vi "OP500Z8_PV generator OP100ZENPlus.vi"(6 "3P4S?":bool, 8 "errin":errorcluster, 10 "network":path, 11 "path in":path) -> (0 "sortie d'erreur":errorcluster caption="errout", 2 "network out":path, 3 "tout bon":bool)   [LabVIEW 2020]
uses:
  <vilib>/regexp/Match Regular Expression.xnode
panel:
  out "nombre de remplacements":i32
  out "Chaîne":string
  out "tableau":string[][](array[string])
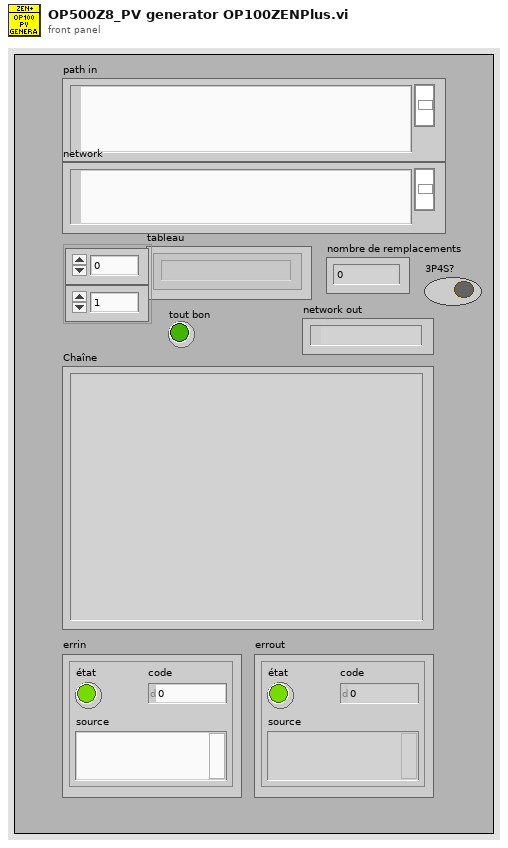
[diagram p1: front panel]
types:
  T1 = enum16{"open", "replace", "create", "open or create", "replace or create", "replace or create with confirmation"}
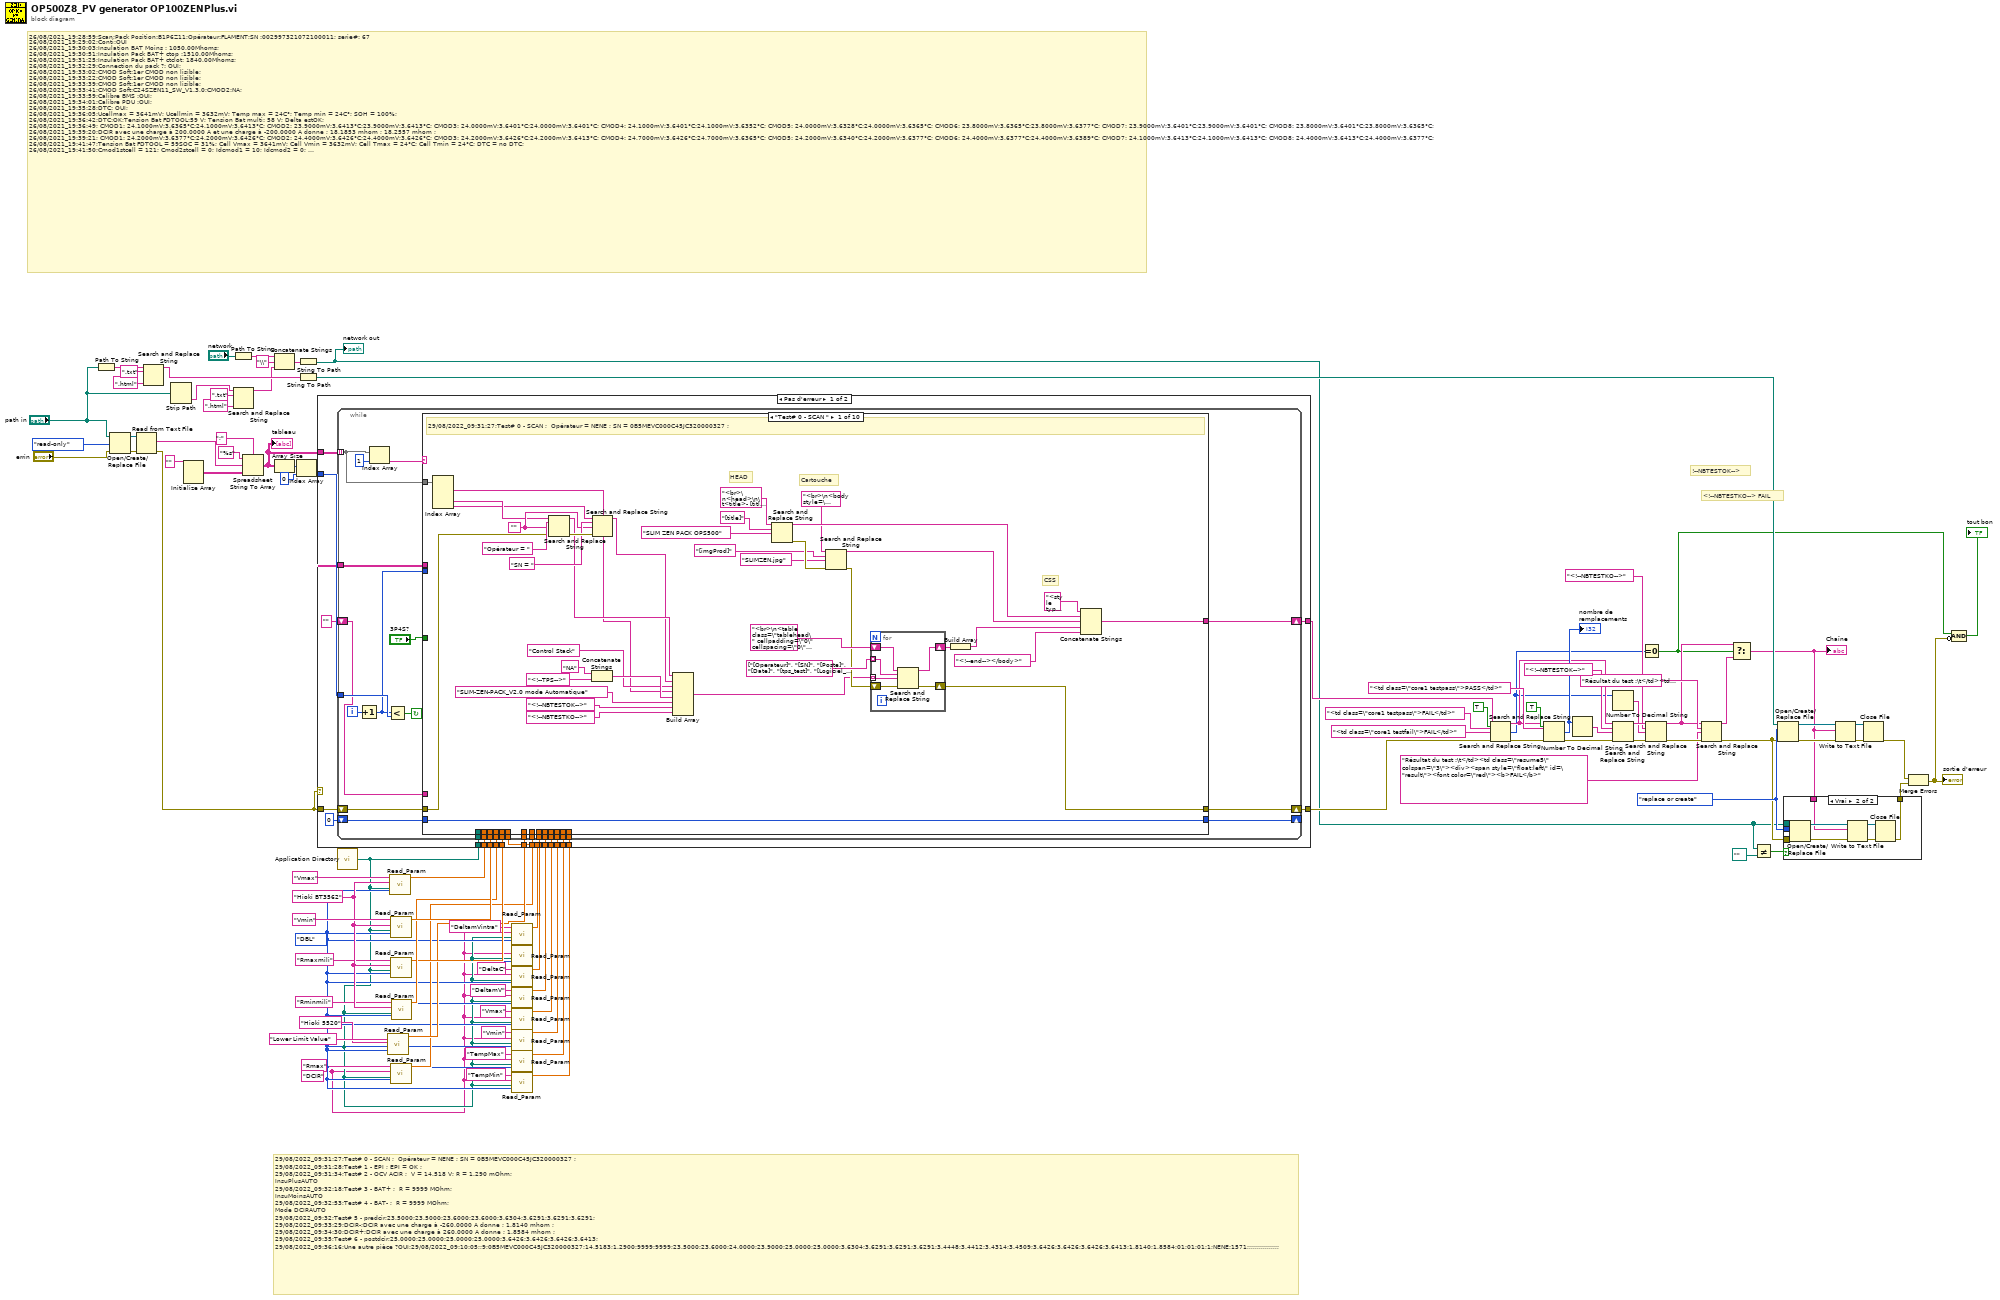
[diagram p0: block diagram]
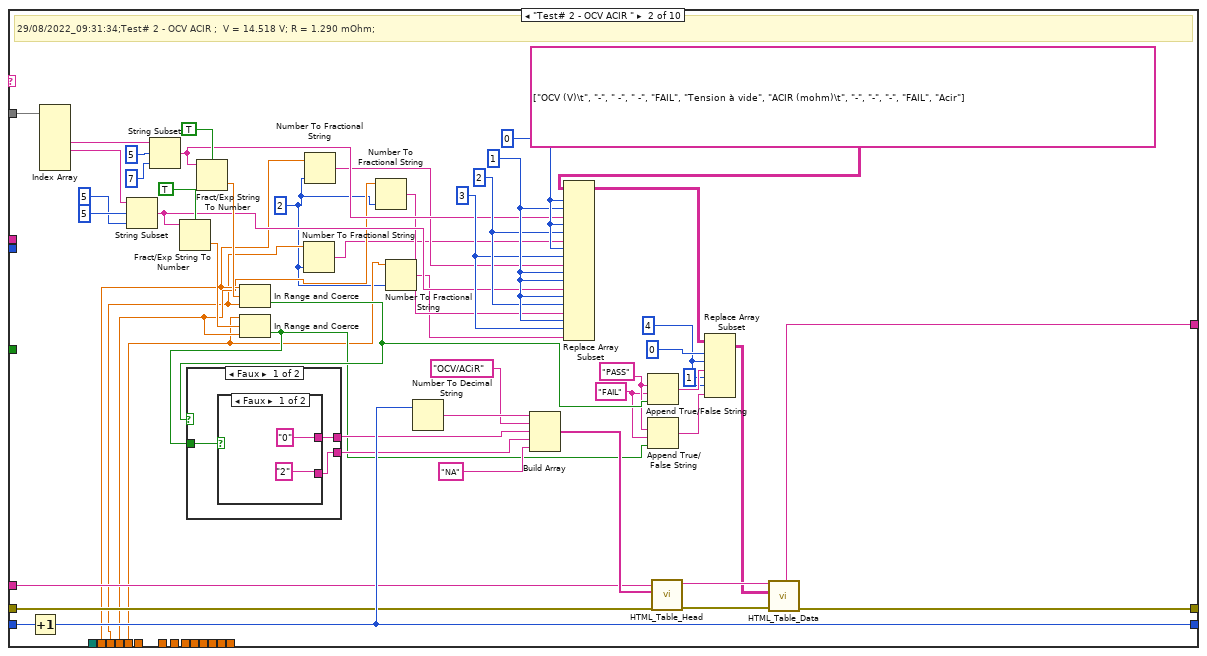
[diagram p2: hidden frame]
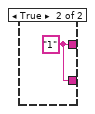
[diagram p3: hidden frame]
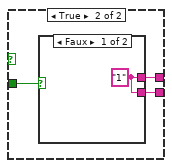
[diagram p4: hidden frame]
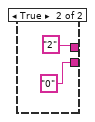
[diagram p5: hidden frame]
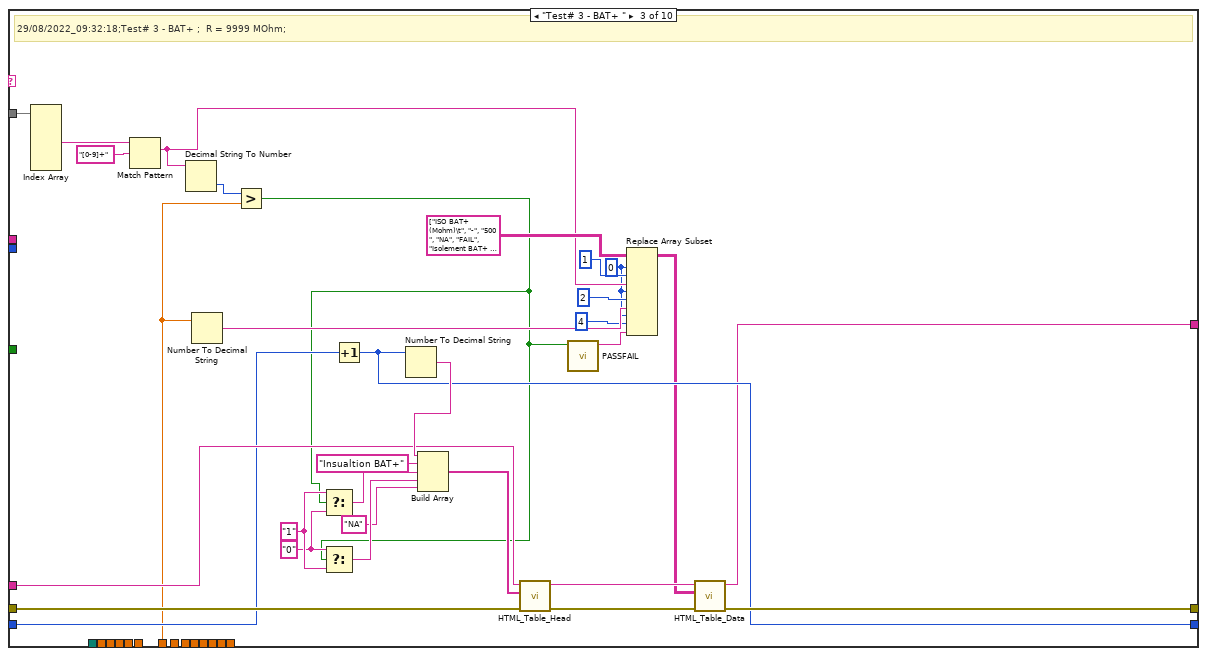
[diagram p6: hidden frame]
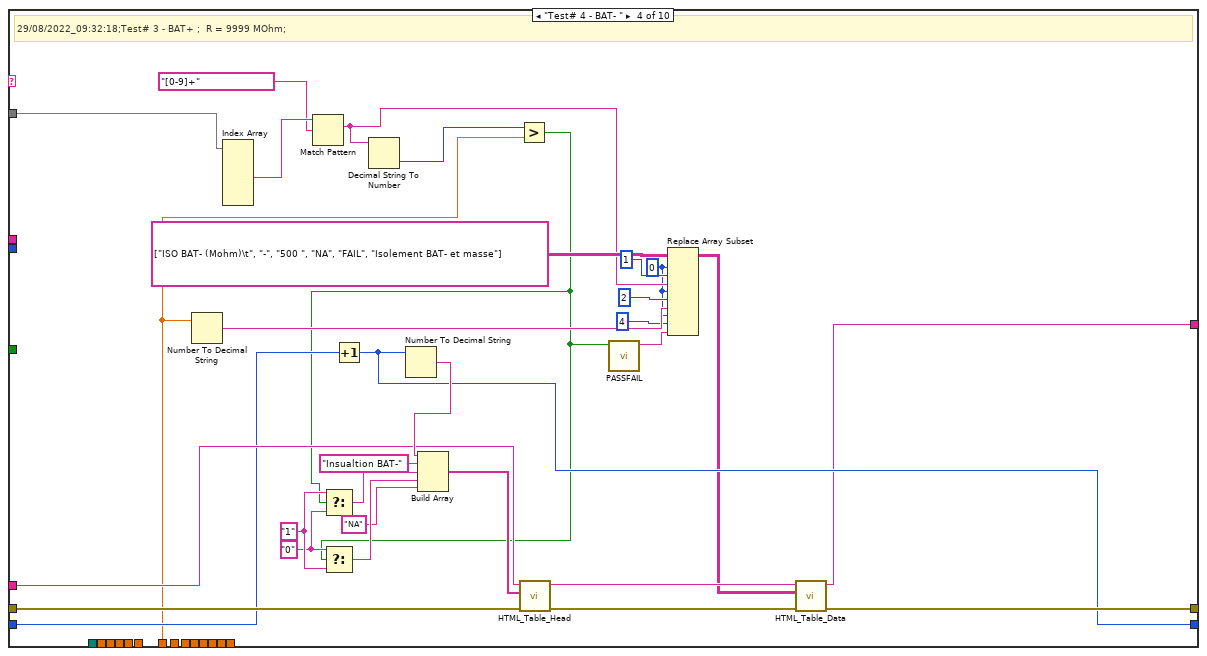
[diagram p7: hidden frame]
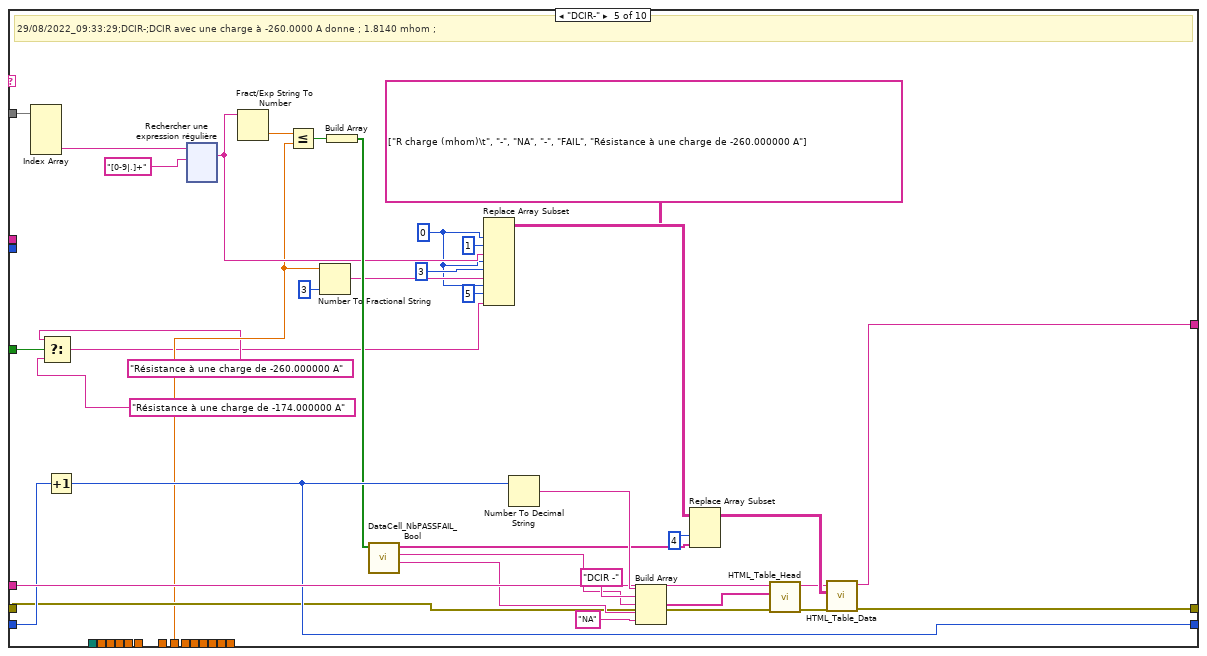
[diagram p8: hidden frame]
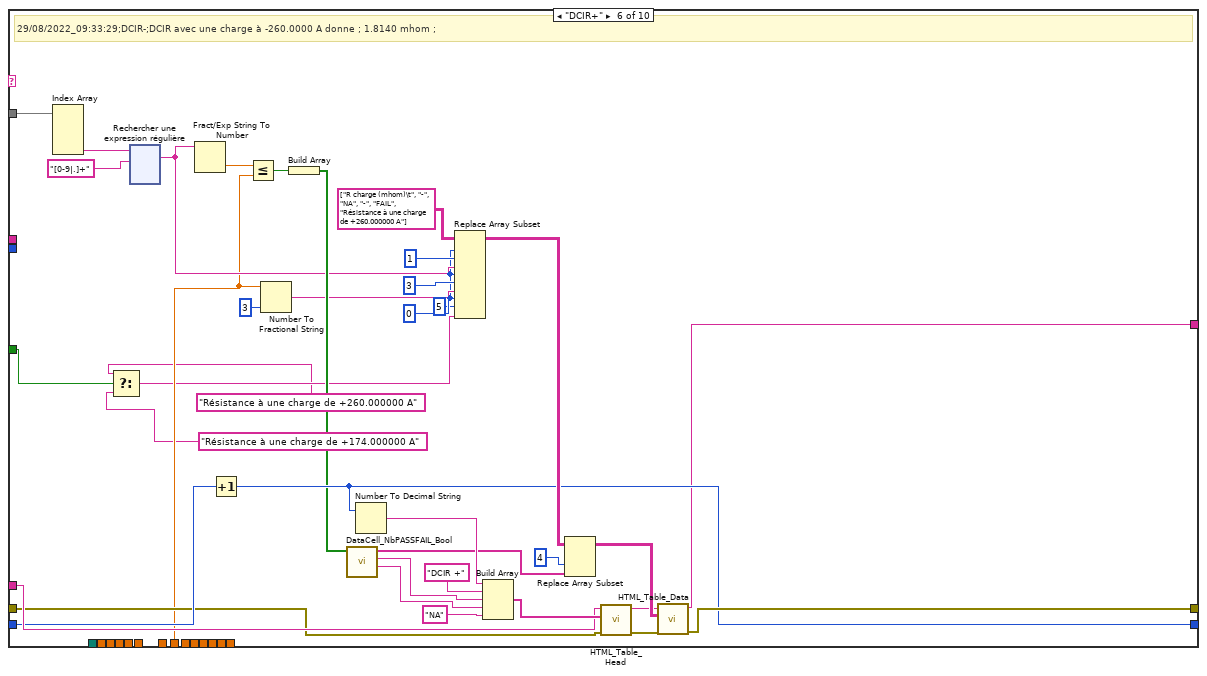
[diagram p9: hidden frame]
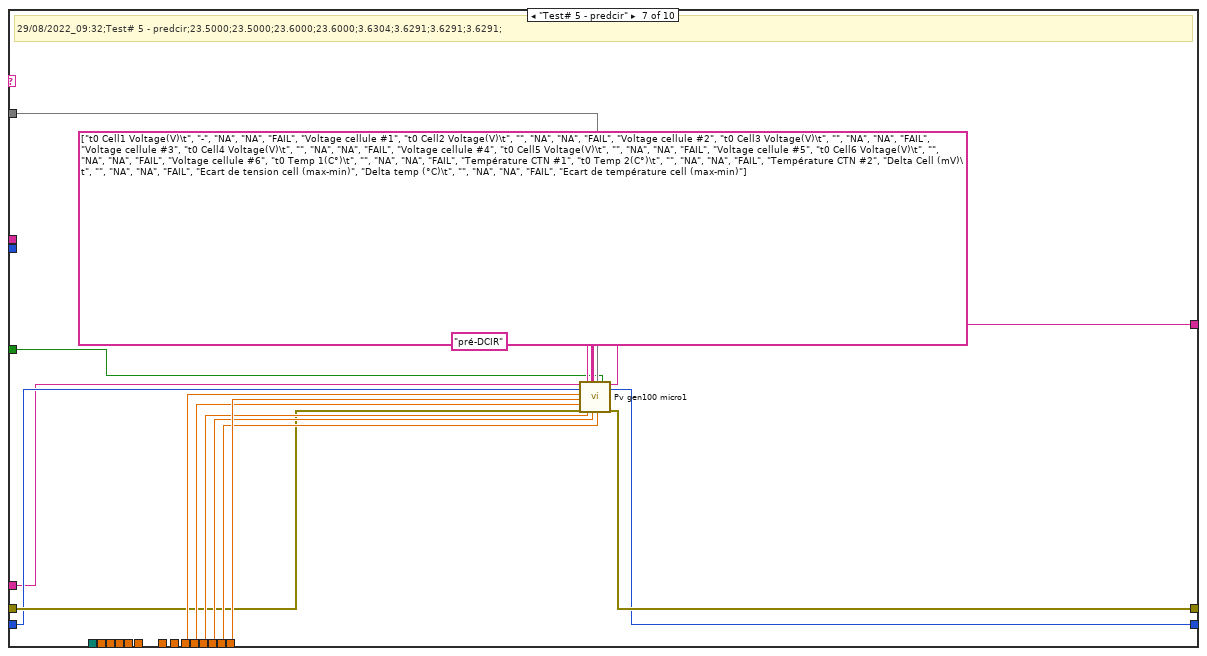
[diagram p10: hidden frame]
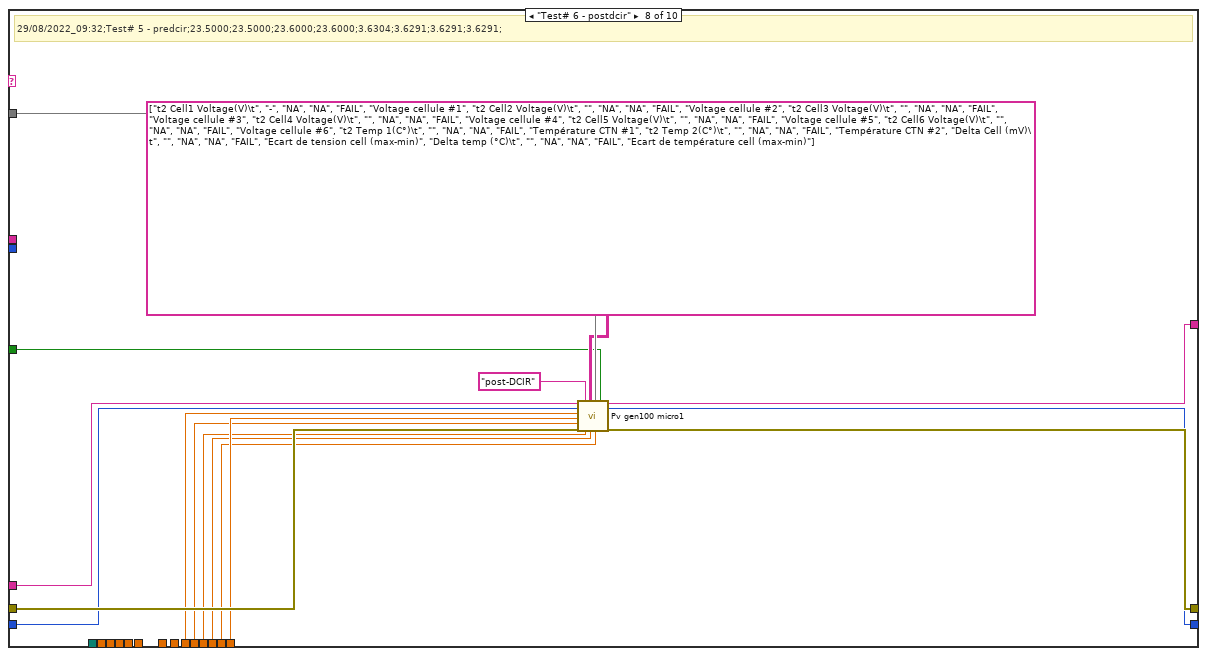
[diagram p11: hidden frame]
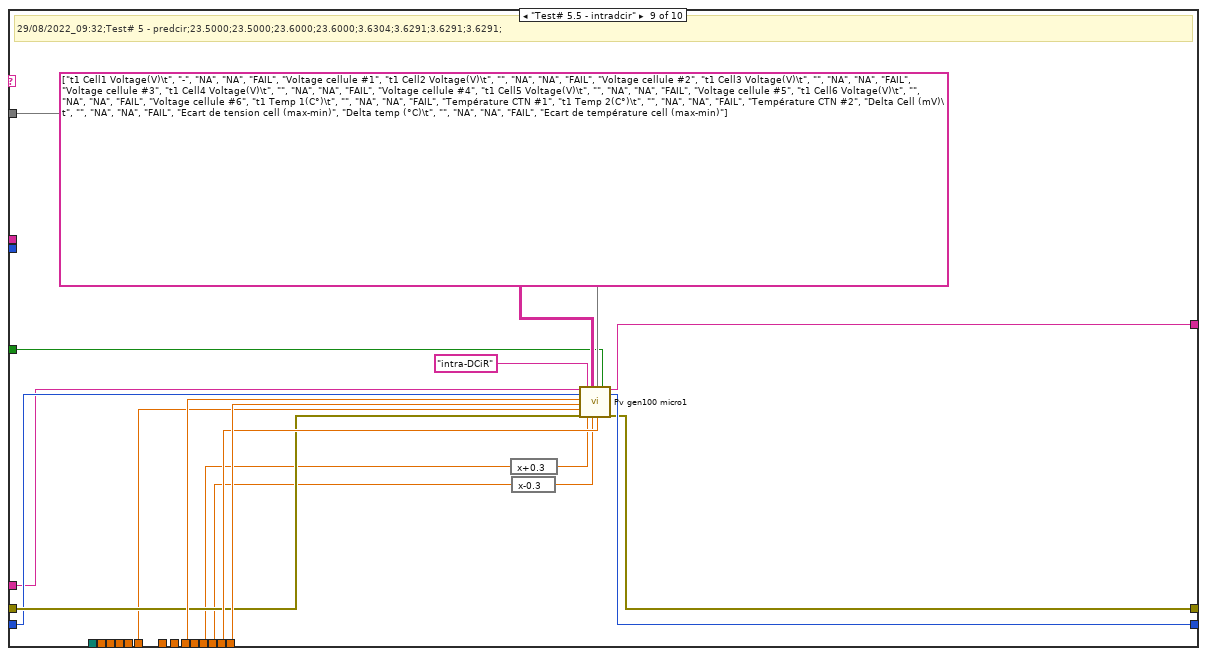
[diagram p12: hidden frame]
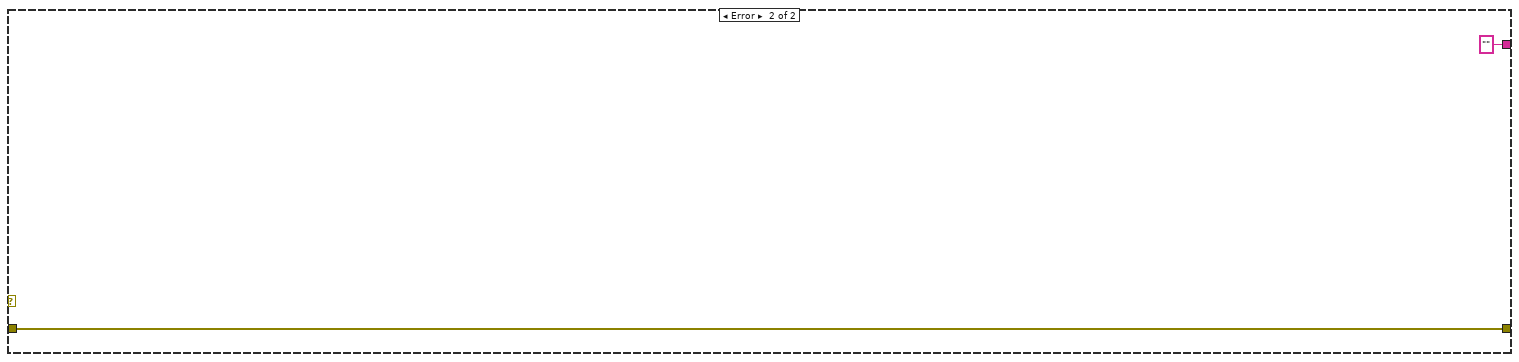
[diagram p14: hidden frame]
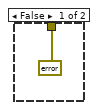
[diagram p15: hidden frame]
diagram:
  w30 = "DCIR" ("section")
  w32 = enum16{"STR", "DBL", "U32"}."DBL" ("Énum")
  w44 = "Hioki BT3562" ("key")
  w58 = T1."replace or create" ("opération (0 : open)")
  # "29/08/2022_09:31:27;Test# 0 - SCAN ;  Opérateur = NENE ; SN = 0B5MEVC000C45JC320000327 ;\n29/08/2022_09:31:28;Test# 1 - EPI ; EPI = OK ;\n29/08/2022_09:31:34;Test# 2 - OCV ACIR ;  V = 14.518 V; R = 1.290 mOhm;\nInsuPlusAUTO\n29/08/2022_09:32:18;Test# 3 - BAT+ ;  R = 9999 MOhm;\nInsuMoinsAUTO\n29/08/2022_09:32:53;Test# 4 - BAT- ;  R = 9999 MOhm;\nMode DCIRAUTO\n29/08/2022_09:32;Test# 5 - predcir;23.5000;23.5000;23.6000;23.6000;3.6304;3.6291;3.6291;3.6291;\n29/08/2022_09:33:29;DCIR-;DCIR avec une charge à -260.0000 A donne ; 1.8140 mhom ; \n29/08/2022_09:34:30;DCIR+;DCIR avec une charge à 260.0000 A donne ; 1.8584 mhom ; \n29/08/2022_09:35;Test# 6 - postdcir;25.0000;25.0000;25.0000;25.0000;3.6426;3.6426;3.6426;3.6413;\n29/08/2022_09:36:16;Une autre pièce ?OUI;29/08/2022_09:10:05;;9;0B5MEVC000C45JC320000327;14.5183;1.2900;9999;9999;23.5000;23.6000;24.0000;23.9000;25.0000;25.0000;3.6304;3.6291;3.6291;3.6291;3.4448;3.4412;3.4314;3.4509;3.6426;3.6426;3.6426;3.6413;1.8140;1.8584;01;01;01;1;NENE;1571;;;;;;;;;;;;;;;;"
  # "<!--NBTESTKO--> FAIL"
  # "!--NBTESTOK-->"
  # "26/08/2021_19:28:59;Scan;Pack Position:B1P6Z11;Opérateur:FLAMENT;SN :002997321072100011; serie#: 67\n26/08/2021_19:29:02;Conti:OUI\n26/08/2021_19:30:03;Insulation BAT Moins : 1050.00Mhoms;\n26/08/2021_19:30:51;Insulation Pack BAT+ ctop :1510.00Mhoms;\n26/08/2021_19:31:25;Insulation Pack BAT+ ctclot: 1840.00Mhoms;\n26/08/2021_19:32:29;Connection du pack ?: OUI;\n26/08/2021_19:33:02;CMOD Soft:1er CMOD non lisible;\n26/08/2021_19:33:22;CMOD Soft:1er CMOD non lisible;\n26/08/2021_19:33:39;CMOD Soft:1er CMOD non lisible;\n26/08/2021_19:33:41;CMOD Soft:C24SZEN11_SW_V1.3.0;CMOD2:NA;\n26/08/2021_19:33:59;Calibre BMS :OUI;\n26/08/2021_19:34:01;Calibre PDU :OUI;\n26/08/2021_19:35:28;DTC: OUI;\n26/08/2021_19:36:05;Ucellmax = 3641mV; Ucellmin = 3632mV; Temp max = 24C°; Temp min = 24C°; SOH = 100%;\n26/08/2021_19:36:42;DTC:OK;Tension Bat FDTOOL:59 V; Tension Bat multi: 58 V; Delta estOK;\n26/08/2021_19:36:49; CMOD1: 24.1000mV;3.6365°C;24.1000mV;3.6413°C; CMOD2: 23.9000mV;3.6413°C;23.9000mV;3.6413°C; CMOD3: 24.0000mV;3.6401°C;24.0000mV;3.6401°C; CMOD4: 24.1000mV;3.6401°C;24.1000mV;3.6352°C; CMOD5: 24.0000mV;3.6328°C;24.0000mV;3.6365°C; CMOD6: 23.8000mV;3.6365°C;23.8000mV;3.6377°C; CMOD7: 23.9000mV;3.6401°C;23.9000mV;3.6401°C; CMOD8: 23.8000mV;3.6401°C;23.8000mV;3.6365°C;\n26/08/2021_19:39:20;DCIR avec une charge à 200.0000 A et une charge à -200.0000 A donne ; 18.1853 mhom ; 18.2557 mhom ; \n26/08/2021_19:39:21; CMOD1: 24.2000mV;3.6377°C;24.2000mV;3.6426°C; CMOD2: 24.4000mV;3.6426°C;24.4000mV;3.6426°C; CMOD3: 24.2000mV;3.6426°C;24.2000mV;3.6413°C; CMOD4: 24.7000mV;3.6426°C;24.7000mV;3.6365°C; CMOD5: 24.2000mV;3.6340°C;24.2000mV;3.6377°C; CMOD6: 24.4000mV;3.6377°C;24.4000mV;3.6389°C; CMOD7: 24.1000mV;3.6413°C;24.1000mV;3.6413°C; CMOD8: 24.4000mV;3.6413°C;24.4000mV;3.6377°C;\n26/08/2021_19:41:47;Tension Bat FDTOOL = 59SOC = 31%; Cell Vmax = 3641mV; Cell Vmin = 3632mV; Cell Tmax = 24°C; Cell Tmin = 24°C; DTC = no DTC;\n26/08/2021_19:41:50;Cmod1stcell = 121; Cmod2stcell = 0; Idcmod1 = 10; Idcmod2 = 0; ReId = KO;\n26/08/2021_19:42:38;Next ? PAS OK"
  n1 = Path To String(path="path in") -> (string=w80:string)
  n2 = Open/Create/Replace File(file path (use dialog)="path in", error in="errin", access (0:read/write)=enum16{"read/write", "read-only", "write-only"}."read-only" ("accès (0 : read/write)")) -> (refnum out=w81:refnum<file>, error out=w96:errorcluster)  [unwired: 3 in, 1 out]
  n3 = Read from Text File(file (use dialog)=w81, error in=w96) -> (text=w92:string, error out=w1:errorcluster)  [unwired: 2 in, 2 out]
  n4 = Search and Replace String(input string=w80, search string=".txt" ("chaîne recherchée"), replace string=".html" ("chaîne de remplacement (\"\")")) -> (result string=w77:string)  [unwired: 5 in, 3 out]
  n5 = Strip Path(path="path in") -> (name=w8:string)  [unwired: 1 out]
  n6 = Initialize Array("") -> (w94:string[][])  [unwired: 2 in]
  n7 = Path To String(path="network") -> (string=w7:string)
  n8 = Search and Replace String(input string=w8, search string=".txt" ("chaîne recherchée"), replace string=".html" ("chaîne de remplacement (\"\")")) -> (result string=w5:string)  [unwired: 5 in, 3 out]
  n9 = Spreadsheet String To Array(delimiter (Tab)=";" ("séparateur (Tabulation)"), format string="%s" ("chaîne de format"), spreadsheet string=w92, array type (2D Dbl)=w94) -> (array=w87:string[][])
  "tableau" <- w87
  n10 = Concatenate Strings(w7, "\\" ("chaîne"), w5) -> (w4:string)
  n11 = Array Size(array=w87) -> (size(s)=w90:i32[])
  n12 = Index Array(array=w90, index=0 ("indice")) -> (element=w88:i32)
  n13 = String To Path(string=w4) -> (path=w10:path)
  "network out" <- w10
  n14 = String To Path(string=w77) -> (path=w76:path)
  n15 = call <vilib>:"Application Directory.vi"() -> ("Application Directory"=w31:path)
  n16 = call <userlib>:"Read_Param.vi"("Énum"=w32, "pathin"=w31, "section"="Hioki 5520", "key"="Lower Limit Value") -> ("dbl"=w36:dbl)  [unwired: 4 in, 3 out]
  n17 = call <userlib>:"Read_Param.vi"("Énum"=w32, "pathin"=w31, "section"=w44, "key"="Vmax") -> ("dbl"=w41:dbl)  [unwired: 4 in, 3 out]
  n18 = call <userlib>:"Read_Param.vi"("Énum"=w32, "pathin"=w31, "section"=w44, "key"="Vmin") -> ("dbl"=w40:dbl)  [unwired: 4 in, 3 out]
  n19 = call <userlib>:"Read_Param.vi"("Énum"=w32, "pathin"=w31, "section"=w44, "key"="Rmaxmili") -> ("dbl"=w38:dbl)  [unwired: 4 in, 3 out]
  n20 = call <userlib>:"Read_Param.vi"("Énum"=w32, "pathin"=w31, "section"=w30, "key"="Rmax") -> ("dbl"=w33:dbl)  [unwired: 4 in, 3 out]
  n21 = call <userlib>:"Read_Param.vi"("Énum"=w32, "pathin"=w31, "section"=w44, "key"="Rminmili") -> ("dbl"=w39:dbl)  [unwired: 4 in, 3 out]
  n22 = call <userlib>:"Read_Param.vi"("Énum"=w32, "pathin"=w31, "section"=w30, "key"="DeltamVintra") -> ("dbl"=w2:dbl)  [unwired: 4 in, 3 out]
  n23 = call <userlib>:"Read_Param.vi"("Énum"=w32, "pathin"=w31, "section"=w30) -> ()  [unwired: 5 in, 4 out]
  n24 = call <userlib>:"Read_Param.vi"("Énum"=w32, "pathin"=w31, "section"=w30, "key"="DeltaC") -> ("dbl"=w23:dbl)  [unwired: 4 in, 3 out]
  n25 = call <userlib>:"Read_Param.vi"("Énum"=w32, "pathin"=w31, "section"=w30, "key"="DeltamV") -> ("dbl"=w22:dbl)  [unwired: 4 in, 3 out]
  n26 = call <userlib>:"Read_Param.vi"("Énum"=w32, "pathin"=w31, "section"=w30, "key"="Vmax") -> ("dbl"=w21:dbl)  [unwired: 4 in, 3 out]
  n27 = call <userlib>:"Read_Param.vi"("Énum"=w32, "pathin"=w31, "section"=w30, "key"="Vmin") -> ("dbl"=w20:dbl)  [unwired: 4 in, 3 out]
  n28 = call <userlib>:"Read_Param.vi"("Énum"=w32, "pathin"=w31, "section"=w30, "key"="TempMax") -> ("dbl"=w19:dbl)  [unwired: 4 in, 3 out]
  n29 = call <userlib>:"Read_Param.vi"("Énum"=w32, "pathin"=w31, "section"=w30, "key"="TempMin") -> ("dbl"=w18:dbl)  [unwired: 4 in, 3 out]
  n30 = case shown="Pas d'erreur" w1 {
    tunnel: w88 -> [w118 _]
    tunnel: w87 -> [w116 _]
    tunnel: w1 -> [w114 w674]
    tunnel: [w113 ""] -> w75
    tunnel: [w112 w674] -> w73
    tunnel: w41 -> [w111 _]
    tunnel: w40 -> [w110 _]
    tunnel: w39 -> [w109 _]
    tunnel: w38 -> [w108 _]
    tunnel: w36 -> [w107 _]
    tunnel: w33 -> [w106 _]
    tunnel: w31 -> [w105 _]
    tunnel: w23 -> [w104 _]
    tunnel: w22 -> [w103 _]
    tunnel: w21 -> [w102 _]
    tunnel: w20 -> [w101 _]
    tunnel: w19 -> [w100 _]
    tunnel: w18 -> [w99 _]
    tunnel: w2 -> [w98 _]
    frame No Error {
      n31 = while {
        tunnel: w118 -> [w146]
        tunnel: w116 -> [w142] mode=indexing
        shift-right: [w141] -> w112
        shift-left: w114 -> [w140]
        shift-right: [w134] -> w113
        shift-left: "" -> [w139]
        shift-right: [w137] -> _
        shift-left: 0 -> [w138]
        tunnel: w116 -> [w136]
        tunnel: w105 -> [w133]
        tunnel: w111 -> [w132]
        tunnel: w110 -> [w131]
        tunnel: w109 -> [w130]
        tunnel: w108 -> [w129]
        tunnel: w107 -> [w128]
        tunnel: w106 -> [w127]
        tunnel: w104 -> [w126]
        tunnel: w103 -> [w125]
        tunnel: w102 -> [w124]
        tunnel: w101 -> [w123]
        tunnel: w100 -> [w122]
        tunnel: w99 -> [w121]
        tunnel: w98 -> [w119]
        i -> [w147]
        stop <- w145 continue-if-true
        n32 = Increment(x=w147) -> (x+1=w135:i32)
        n33 = Index Array(array=w142, index=1 ("indice")) -> (element=w143:string)
        n34 = Less?(x=w135, y=w146) -> (x < y?=w145:bool)
        n35 = case shown="\"Test# 0 - SCAN \"" w143 {
          tunnel: w140 -> [w183 w230 w273 w304 w332 w483 w629 w649 w666 w672]
          tunnel: w142 -> [w185 w238 w274 w305 w341 w492 w623 w645 w662 _]
          tunnel: [w153 w229 w272 w303 w344 w495 w628 w648 w659 w672] -> w141
          tunnel: w139 -> [_ w228 w271 w302 w345 w496 w621 w650 w664 w670]
          tunnel: w138 -> [w152 w243 w270 w301 w343 w494 w622 w647 w665 w671]
          tunnel: [w152 w237 w269 w300 w342 w493 w627 w646 w660 w671] -> w137
          tunnel: w136 -> [_ _ _ _ _ _ _ _ _ _]
          tunnel: w135 -> [_ _ _ _ _ _ _ _ _ _]
          tunnel: [w151 w226 w268 w299 w335 w486 w626 w644 w661 w670] -> w134
          tunnel: w133 -> [_ _ _ _ _ _ _ _ _ _]
          tunnel: w132 -> [_ w200 _ _ _ _ _ _ _ _]
          tunnel: w131 -> [_ w195 _ _ _ _ _ _ _ _]
          tunnel: w130 -> [_ w198 _ _ _ _ _ _ _ _]
          tunnel: w129 -> [_ w193 _ _ _ _ _ _ _ _]
          tunnel: w128 -> [_ _ w257 w288 _ _ _ _ _ _]
          tunnel: w127 -> [_ _ _ _ w326 w477 _ _ _ _]
          tunnel: w126 -> [_ _ _ _ _ _ w630 w639 w667 _]
          tunnel: w125 -> [_ _ _ _ _ _ w631 w638 _ _]
          tunnel: w124 -> [_ _ _ _ _ _ w632 w640 w655 _]
          tunnel: w123 -> [_ _ _ _ _ _ w633 w641 w656 _]
          tunnel: w122 -> [_ _ _ _ _ _ w634 w642 w668 _]
          tunnel: w121 -> [_ _ _ _ _ _ w635 w643 w669 _]
          tunnel: "3P4S?" -> [_ _ _ _ w323 w470 w620 w636 w653 _]
          tunnel: w119 -> [_ _ _ _ _ _ _ _ w652 _]
          frame "Test# 0 - SCAN " {
            w155 = ""
            # "Cartouche"
            # "HEAD"
            # "CSS"
            # "29/08/2022_09:31:27;Test# 0 - SCAN ;  Opérateur = NENE ; SN = 0B5MEVC000C45JC320000327 ;"
            n36 = Index Array(array=w185) -> (element #1=w154:string, element #3=w150:string, element #4=w148:string)  [unwired: 4 in, 1 out]
            n37 = Search and Replace String(input string=w150, search string="Opérateur = " ("chaîne recherchée"), replace string=w155, error in=w183) -> (result string=w156:string, error out=w182:errorcluster)  [unwired: 4 in, 2 out]
            n38 = Concatenate Strings("NA" ("chaîne"), "<!--TPS-->" ("chaîne")) -> (w161:string)
            n39 = Search and Replace String(input string=w148, search string="SN = ", replace string=w155, error in=w182) -> (result string=w149:string)  [unwired: 4 in, 3 out]
            n40 = Build Array(w156, w149, "Control Stack" ("chaîne"), w154, w161, "SLIM-ZEN-PACK_V2.0 mode Automatique" ("chaîne"), "<!--NBTESTOK-->" ("chaîne"), "<!--NBTESTKO-->" ("chaîne")) -> (w157:string[])
            n41 = Search and Replace String(input string="<br>\n<head>\n\t<title>- [title] -</title>\n</head>", search string="[title]" ("chaîne recherchée"), replace string="SLIM ZEN PACK OPS500" ("Title")) -> (result string=w177:string, error out=w176:errorcluster)  [unwired: 5 in, 2 out]
            n42 = Search and Replace String(input string="<br>\n<body style=\"text-align: center;\" onload=\"InitInterface();\">\n\n<table class=\"tablehead resume0\">\n\t<tbody>\n\t\t<tr>\n\t\t\t<td> <img src=\"[imgProd]\" style=\"width:194px;height:100px\" class=\"left\"></td>\n\t\t\t<td> <div class=\"center\">PROCES VERBAL DE TEST AUTOMATIQUE</div><br class=\"center\"><div class=\"center\">Forseepower</div></td>\n\t\t\t<td> <img src=\"LOGO FORSEE.png\" style=\"width:194px;height:100px\"  class=\"right\"></td>\n\t\t</tr>\n\t</tbody>\n</table>", search string="[imgProd]", replace string="SLIMZEN.jpg" ("imgProd"), error in=w176) -> (result string=w173:string, error out=w170:errorcluster)  [unwired: 4 in, 2 out]
            n43 = for {
              shift-right: [w190] -> w169
              shift-left: "<br>\n<table class=\"tablehead\" cellpadding=\"0\" cellspacing=\"0\">\n\t<tbody>\n\t\t<tr><td class=\"resume3\">Opérateur :\t</td><td class=\"resume5\" colspan=\"3\">[Operateur]</td></tr>\n\t\t<tr><td class=\"resume3\">SN : </td><td class=\"resume5\" colspan=\"3\">[SN]</td></tr>\n\t\t<tr><td class=\"resume3\">Poste : </td><td class=\"resume5\" colspan=\"3\">[Poste]</td></tr>\t\t\n\t\t<tr><td class=\"resume3\">Date du test : </td><td class=\"resume5\" colspan=\"3\">[Date]</td></tr>\n\t\t<tr><td class=\"resume3\">Temps de test : </td><td class=\"resume5\" colspan=\"3\">[tps_test]</td></tr>\n\t\t<tr><td class=\"resume3\">Logiciel de test :\t</td><td class=\"resume5\" colspan=\"3\">[Logiciel_test]</td></tr>\n\t\t<tr><td class=\"resume3\">Résultat du test :\t</td><td class=\"resume5\" colspan=\"3\"><div><span style=\"float:left\" id=\"result\"><font color=\"green\"><b>PASS</b></font><b> ( <font color=\"green\">[NbPASS] PASS</font> / <font color=\"red\">[NbFAIL] FAIL</font> )</b></span></div></td></tr>\n\t</tbody>\n</table>" -> [w191]
              tunnel: string[] ["[Operateur]", "[SN]", "[Poste]", "[Date]", "[tps_test]", "[Logiciel_test]", "[NbPASS]", "[NbFAIL]"] -> [w187] mode=indexing
              tunnel: w157 -> [w186] mode=indexing
              shift-right: [w188] -> w153
              shift-left: w170 -> [w189]
              n44 = Search and Replace String(input string=w191, search string=w187, replace string=w186, error in=w189) -> (result string=w190:string, error out=w188:errorcluster)  [unwired: 4 in, 2 out]
            }
            n45 = Build Array(w169) -> (w168:string[])
            n46 = Concatenate Strings("<style type=\"text/css\">\n\n.resume1,.resume3,.resume4,.resume5,.resume6,.resume7{background-color:#e6feef;padding:7px;border:1px solid black;}\n.resume0{border:1px solid black;background-color:#e6feef;font-weight: bold;padding:0px;text-align: center;}\n.resume1{width:350px;text-align:right;font-weight:bold;}\n.resume3{width:350px;text-align:right;border-top:0px solid black;font-weight:bold;}\n.resume4{border-left:0px solid black;width:290px;}\n.resume5{width:290px;border-left:0px solid black;border-top:0px solid black;}\n.resume6{border-left:0px solid black;width:60px;}\n.resume7{border-left:0px solid black;border-top:0px solid black;width:60px;}\n.title1{text-align: left;background-color:#e6f4fe;padding:10px;border:1px solid #101010;}\n.title2{width: 30px;text-align: center;background-color:#e6f4fe;padding:1px;border:1px solid #101010;border-left:0px solid black;font-weight: bold;}\n.title2 a:link{text-decoration:none;}\n.entete0,.entete1,.entete2,.time2{text-align: center;background-color:#feeec9;padding:7px;border:1px solid black;font-weight: bold;}\n.entete0{width:45px;border-right:0px solid black;}\n.entete1{width:505px;}\n.entete2{width:95px;border-right:0px solid black;}\n.time2{border-left:0px solid black;width:145px;font-size:11px;}\n.core0,.core1,.core2,.core3,.core4,.time{text-align: center;background-color:#fafed3;padding:7px;border:1px solid black;}\n.core0, .core1,.core3,.core4{width:95px;border-top:0px solid black;border-right:0px solid black;}\n.core0{width:45px;}\n.core2{border-top:0px solid black;width:505px;}\n.core3{width:200px;}\n.core4{width:300px;}\n.time{width:145px;border-top:0px solid black;border-left:0px solid black;font-size:11px;}\n.false .core0,.false .core1,.false .core2,.false .core3,.false .core4,.false .time{background-color:#f4f4f4;}\n.false .entete0,.false .entete1,.false .entete2,.false .time2{background-color:#dadada;}\n.false .title1,.false .title2,.false .resultentete .testpass,.false .resultentete .testfail,.false .resultentete .testtime{background-color:#c5cac9;color: blue;}\n.false .title2 a:link{text-decoration:none;color: blue;}\n.comment1,.comment2,.time3{width: 890px;background-color:#e9e8e9;padding:7px;border:1px solid black;border-top:0px solid black;text-align:left;}\n.comment2{border-right:0px solid black;width: 45px;text-align: center;}\n.time3{width: 145px;border-left:0px solid black;font-size:11px;}\n.fixe1{background: -moz-linear-gradient(center top , #101010 10%, #555555 80%) repeat scroll 0 0 transparent;background: -webkit-gradient(linear, left top, left bottom, from(#101010), to(#555555));border:2px solid orange;position : fixed;margin-top:20px;display:none;overflow-y:scroll;max-height:350px;text-shadow: 0px 0px 0 #333333;text-align:left;font-size:10px;padding:10px;margin-left:-162px;border-radius: 15px 15px 15px 15px;}\n.menufixe, .menufixelock{background: -moz-linear-gradient(center top , #101010 80%, transparent 20%) repeat scroll 0 0 transparent;background: -webkit-gradient(linear, left top, left bottom, from(#101010), color-stop(0.65, #101010), to(transparent)) repeat scroll 0 0 transparent;margin: -52px 0px 0px -9px;width:100%;position:fixed;height:55px;-moz-transition: margin 1s;-webkit-transition: margin 1s;}\n.menufixelock, .menufixe:hover{margin: -9px 0px 0px -9px;}\n.lockmenu, .separation,.separationmenu{text-align:center;background: -moz-linear-gradient(center top , #555555 10%, #111111 80%) repeat scroll 0 0 transparent;background: -webkit-gradient(linear, left top, left bottom, from(#555555), to(#111111));border: 1px solid white;border-radius: 10px 10px 10px 10px;box-shadow: 0 -1px 1px #555555 inset;color: #999999;font-weight: bold;width: 100px;padding: 2px;text-decoration: none;}\n.tablehead{width: 1000px;font-family: Verdana;font-size: 12px;margin-left: auto;margin-right: auto;}\n.tablenull{font-family: Verdana;font-size: 11px;margin-left: auto;margin-right: auto;}\n.separationmenu:hover div{display: inline;}\n.lockmenu:hover, .separation:hover,.separationmenu:hover{border: 1px solid orange;cursor:pointer;}\n.lockmenu:hover{border: 1px solid red;cursor:pointer;}\n.separationright{padding:10px;}\ndiv a:link{text-decoration:none;color:#cbcbcb;}\ndiv a:hover{text-decoration:underline;color:#cbcbcb;}\nspan a:link{text-decoration:none;color:#cbcbcb;}\nspan a:hover{text-decoration:none;color:#cbcbcb;}\n.false{color: blue;}\n.testpass{color: green;font-weight: bold;}\n.testfail{color: red;font-weight: bold;}\n.testtime{color: blue;font-weight: bold;}\n.resultentete{font-weight: bold;font-size: 11px;min-width: 200px;text-align:right;}\n.infohard{border: 1px solid black;background-color: white;text-align: center;width: 16px;height: 16px;border-radius: 5px;font-weight: bold;box-shadow: 0 -1px 2px #555555 inset;}\n.infohard:hover{background-color:#feeec9;cursor:pointer;}\n.footerhard{padding-top:30px;}\n.confighard{font-size:10px;width:110px;}\n.circlemain{margin-left:auto;margin-right:auto;}\n.circletext,.circleform{padding-top: 3px;text-align:center;font-size: 10px;width:200px;}\n.circleform{padding-bottom: 3px;padding-top: 1px;}\n.circle{border: 1px solid black;border-collapse: collapse;border-radius: 15px;box-shadow: 1px 1px 0 #505050;height: 15px;width: 15px;display:inline-block;}\n.bookmarkon, .bookmarkoff{background-color: yellow;border: 1px solid black;border-collapse: collapse;border-radius: 10px 10px 10px 10px;box-shadow: 1px 1px 0 #505050;height: 12px;width: 12px;position: absolute;margin-left:22px;cursor: help;}\n.bookmarkoff{background-color: transparent;border: 1px solid #CECECE;box-shadow: none;cursor: copy;}\n.false .bookmarkoff{background-color: transparent;border: 1px solid #E6E1E1;box-shadow: none;cursor: copy;}\n.bookmarkmaster{height: 15px;margin-right: 12px;width: 60px;}\n.bookmarkmaster:hover .bookmarkprev,.bookmarkmaster:hover .bookmarksuiv{display:block;}\n.bookmarkprev, .bookmarksuiv {cursor: pointer;font-size: 25px;font-weight: bold;margin-top: -10px;position: absolute;display:none;}\n.bookmarkprev{margin-left: 2px;}\n.bookmarksuiv{margin-left: 43px;}\n.plus, .moins{background-color: #F4F4F4;border: 1px solid #848484;border-radius: 20px;color: #848484;font-family: arial;font-size: 16px;font-weight: bold;height: 20px;margin-left: 4px;text-align: center;width: 20px;}\n.moins{font-size: 15px;}\n.plus:hover, .moins:hover{background-color: #DADADA;border: 1px solid black;color: black;cursor:pointer;}\n.backtothetop {position: fixed; right: 50%; margin-right: -555px; bottom: 10px; font-size: 35px; font-weight: bold; border: 1px solid #7D7B91; width: 40px; height: 40px; line-height:52px; text-align: center;border-radius: 8px; opacity: 0.25; background-color: #F5F5F5; color:#7D7B91;}\n.backtothetop:hover {opacity: 1; cursor:pointer;}\n.libversion {font-size: 8px;font-weight: normal;padding-right: 10px;text-align: right;}\n.lockmenu {width: 18px;font-size: 12px;}\n.left {display: block; margin-left: 1px;margin-right: auto;}\n.right {display: block; margin-right: 1px;margin-left: auto;}\n.center {display: block; margin-left: auto;margin-right: auto;}\n\n</style>", w177, w173, w168, "<!--end--></body>") -> (w151:string)
          }
          frame "Test# 2 - OCV ACIR " {
            w192 = i16 2 ("largeur (-)")
            w209 = 3 ("indice désactivé (col)")
            w210 = 2 ("indice désactivé (col)")
            w212 = 0 ("indice désactivé (ligne)")
            w203 = "FAIL" ("chaîne faux")
            w204 = "PASS" ("chaîne vrai")
            w205 = 4 ("indice désactivé (col)")
            w211 = 1 ("indice désactivé (col)")
            # "29/08/2022_09:31:34;Test# 2 - OCV ACIR ;  V = 14.518 V; R = 1.290 mOhm;"
            n47 = Increment(x=w243) -> (x+1=w237:i32)
            n48 = Index Array(array=w238) -> (element #3=w223:string, element #4=w218:string)  [unwired: 6 in, 4 out]
            n49 = String Subset(string=w218, offset (0)=5, length (rest)=5 ("longueur (reste)")) -> (substring=w207:string)
            n50 = String Subset(string=w223, offset (0)=5, length (rest)=7 ("longueur (reste)")) -> (substring=w208:string)
            n51 = Fract/Exp String To Number(use system decimal point (T)=TRUE ("utiliser le séparateur décimal du système (V)"), string=w207) -> (number=w216:dbl)  [unwired: 2 in, 1 out]
            n52 = Fract/Exp String To Number(use system decimal point (T)=TRUE ("utiliser le séparateur décimal du système (V)"), string=w208) -> (number=w217:dbl)  [unwired: 2 in, 1 out]
            n53 = In Range and Coerce(upper limit=w200, x=w217, lower limit=w195) -> (In Range?=w215:bool)  [unwired: 1 out]
            n54 = In Range and Coerce(upper limit=w193, x=w216, lower limit=w198) -> (In Range?=w202:bool)  [unwired: 1 out]
            n55 = case shown="Faux" w215 {
              tunnel: w202 -> [w246 w252]
              tunnel: [w245 w251] -> w214
              tunnel: [w244 w250] -> w213
              frame False {
                n56 = case shown="Faux" w246 {
                  tunnel: ["0" w249] -> w245
                  tunnel: ["2" w249] -> w244
                  frame False {
                  }
                  frame True {
                    w249 = "1"
                  }
                }
              }
              frame True {
                n57 = case shown="Faux" w252 {
                  tunnel: [w253 "2"] -> w251
                  tunnel: [w253 "0" ("cas faux")] -> w250
                  frame False {
                    w253 = "1"
                  }
                  frame True {
                  }
                }
              }
            }
            n58 = Number To Fractional String(number=w195, precision (6)=w192) -> (F-format string=w196:string)  [unwired: 2 in]
            n59 = Number To Fractional String(number=w200, precision (6)=w192) -> (F-format string=w199:string)  [unwired: 2 in]
            n60 = Number To Fractional String(number=w198, precision (6)=w192) -> (F-format string=w197:string)  [unwired: 2 in]
            n61 = Number To Fractional String(number=w193, precision (6)=w192) -> (F-format string=w194:string)  [unwired: 2 in]
            n62 = Number To Decimal String(number=w237) -> (decimal integer string=w236:string)  [unwired: 1 in]
            n63 = Build Array(w236, "OCV/ACiR" ("élément"), w214, w213, "NA" ("élément")) -> (w241:string[])
            n64 = Replace Array Subset(array=string[][] [["OCV (V)\t", "-", " -", " -", "FAIL", "Tension à vide"], ["ACIR (mohm)\t", "-", "-", "-", "FAIL", "Acir"]] ("Tableau"), new element #1=w208, index (row) #1=w212, index (col) #1=w211, new element #2=w196, index (row) #2=w212, index (col) #2=w210, new element #3=w199, index (row) #3=w212, index (col) #3=w209, new element #4=w207, index (row) #4=w211, index (col) #4=w211, new element #5=w197, index (row) #5=w211, index (col) #5=w210, new element #6=w194, index (row) #6=w211, index (col) #6=w209) -> (w234:string[][])
            n65 = Append True/False String(1:w215, 2:w203, 3:w204) -> (0:w232:string)  [unwired: 1 in]
            n66 = Append True/False String(1:w202, 2:w203, 3:w204) -> (0:w201:string)  [unwired: 1 in]
            n67 = call "HTML_Table_Head.vi"("entrée d'erreur (pas d'erreur)"=w230, "Tableau"=w241, "chaîne en entrée"=w228) -> ("sortie d'erreur"=w240:errorcluster, "result string"=w239:string)  [unwired: 7 in]
            n68 = Replace Array Subset(array=w234, new element #1=w232, index (row) #1=0 ("indice désactivé (ligne)"), index (col) #1=w205, new element #2=w201, index (row) #2=1 ("indice (ligne)"), index (col) #2=w205) -> (w231:string[][])
            n69 = call "HTML_Table_Data.vi"("entrée d'erreur (pas d'erreur)"=w240, "Tableau"=w231, "chaîne en entrée"=w239) -> ("sortie d'erreur"=w229:errorcluster, "result string"=w226:string)  [unwired: 7 in]
          }
          frame "Test# 3 - BAT+ " {
            w262 = 0 ("indice désactivé (ligne)")
            w281 = "0" ("cas faux")
            w282 = "1"
            # "29/08/2022_09:32:18;Test# 3 - BAT+ ;  R = 9999 MOhm;"
            n70 = Index Array(array=w274) -> (element #3=w267:string)  [unwired: 6 in, 5 out]
            n71 = Match Pattern(string=w267, regular expression="[0-9]+" ("chaîne recherchée")) -> (match substring=w265:string)  [unwired: 1 in, 3 out]
            n72 = Decimal String To Number(string=w265) -> (number=w258:i32)  [unwired: 2 in, 1 out]
            n73 = Number To Decimal String(number=w257) -> (decimal integer string=w263:string)  [unwired: 1 in]
            n74 = Greater?(x=w258, y=w257) -> (0:w256:bool)
            n75 = Select(t=w282, s=w256, f=w281) -> (s? t:f=w280:string)
            n76 = Select(t=w281, s=w256, f=w282) -> (s? t:f=w283:string)
            n77 = Increment(x=w270) -> (x+1=w269:i32)
            n78 = Number To Decimal String(number=w269) -> (decimal integer string=w277:string)  [unwired: 1 in]
            n79 = Build Array(w277, "Insualtion BAT+" ("élément"), w280, w283, "NA" ("élément")) -> (w284:string[])
            n80 = call "HTML_Table_Head.vi"("entrée d'erreur (pas d'erreur)"=w273, "Tableau"=w284, "chaîne en entrée"=w271) -> ("sortie d'erreur"=w279:errorcluster, "result string"=w278:string)  [unwired: 7 in]
            n81 = call <userlib>:"PASSFAIL.vi"("E"=w256) -> ("S"=w260:string)  [unwired: 10 in]
            n82 = Replace Array Subset(array=string[][] [["ISO BAT+ (Mohm)\t", "-", "500 ", "NA", "FAIL", "Isolement BAT+ et masse"]] ("Tableau"), new element #1=w265, index (row) #1=w262, index (col) #1=1 ("indice désactivé (col)"), new element #2=w263, index (row) #2=w262, index (col) #2=2 ("indice désactivé (col)"), new element #3=w260, index (row) #3=w262, index (col) #3=4 ("indice désactivé (col)")) -> (w259:string[][])
            n83 = call "HTML_Table_Data.vi"("entrée d'erreur (pas d'erreur)"=w279, "Tableau"=w259, "chaîne en entrée"=w278) -> ("sortie d'erreur"=w272:errorcluster, "result string"=w268:string)  [unwired: 7 in]
          }
          frame "Test# 4 - BAT- " {
            w293 = 0 ("indice désactivé (ligne)")
            w312 = "0" ("cas faux")
            w313 = "1"
            # "29/08/2022_09:32:18;Test# 3 - BAT+ ;  R = 9999 MOhm;"
            n84 = Number To Decimal String(number=w288) -> (decimal integer string=w294:string)  [unwired: 1 in]
            n85 = Index Array(array=w305) -> (element #3=w298:string)  [unwired: 6 in, 5 out]
            n86 = Match Pattern(string=w298, regular expression="[0-9]+" ("chaîne recherchée")) -> (match substring=w296:string)  [unwired: 1 in, 3 out]
            n87 = Increment(x=w301) -> (x+1=w300:i32)
            n88 = Decimal String To Number(string=w296) -> (number=w289:i32)  [unwired: 2 in, 1 out]
            n89 = Number To Decimal String(number=w300) -> (decimal integer string=w308:string)  [unwired: 1 in]
            n90 = Greater?(x=w289, y=w288) -> (0:w287:bool)
            n91 = Select(t=w313, s=w287, f=w312) -> (s? t:f=w311:string)
            n92 = Select(t=w312, s=w287, f=w313) -> (s? t:f=w314:string)
            n93 = Build Array(w308, "Insualtion BAT-" ("élément"), w311, w314, "NA" ("élément")) -> (w315:string[])
            n94 = call "HTML_Table_Head.vi"("entrée d'erreur (pas d'erreur)"=w304, "Tableau"=w315, "chaîne en entrée"=w302) -> ("sortie d'erreur"=w310:errorcluster, "result string"=w309:string)  [unwired: 7 in]
            n95 = call <userlib>:"PASSFAIL.vi"("E"=w287) -> ("S"=w291:string)  [unwired: 10 in]
            n96 = Replace Array Subset(array=string[][] [["ISO BAT- (Mohm)\t", "-", "500 ", "NA", "FAIL", "Isolement BAT- et masse"]] ("Tableau"), new element #1=w296, index (row) #1=w293, index (col) #1=1 ("indice désactivé (col)"), new element #2=w294, index (row) #2=w293, index (col) #2=2 ("indice désactivé (col)"), new element #3=w291, index (row) #3=w293, index (col) #3=4 ("indice désactivé (col)")) -> (w290:string[][])
            n97 = call "HTML_Table_Data.vi"("entrée d'erreur (pas d'erreur)"=w310, "Tableau"=w290, "chaîne en entrée"=w309) -> ("sortie d'erreur"=w303:errorcluster, "result string"=w299:string)  [unwired: 7 in]
          }
          frame "DCIR-" {
            w319 = 0 ("indice désactivé (col)")
            # "29/08/2022_09:33:29;DCIR-;DCIR avec une charge à -260.0000 A donne ; 1.8140 mhom ;"
            n98 = Index Array(array=w341) -> (element #4=w334:string)  [unwired: 4 in, 3 out]
            n99 = Select(t="Résistance à une charge de -260.000000 A", s=w323, f="Résistance à une charge de -174.000000 A") -> (s? t:f=w320:string)
            n100 = Increment(x=w343) -> (x+1=w342:i32)
            n101 = xnode "Rechercher une expression régulière"("chaîne en entrée"=w334, "expression régulière"="[0-9|.]+") -> ("toute l'expression"=w331:string)  [unwired: 4 in, 4 out]
            n102 = Fract/Exp String To Number(string=w331) -> (number=w329:dbl)  [unwired: 3 in, 1 out]
            n103 = Less Or Equal?(x=w329, y=w326) -> (x <= y?=w328:bool)
            n104 = Number To Fractional String(number=w326, precision (6)=i16 3 ("précision (6)")) -> (F-format string=w324:string)  [unwired: 2 in]
            n105 = Build Array(w328) -> (w340:bool[])
            n106 = call <userlib>:"DataCell_NbPASSFAIL_Bool.vi"("Tableau en entrée"=w340) -> ("Chaîne"=w338:string, "Chaîne 2"=w339:string, "Tableau en sortie"=w336:string[])  [unwired: 8 in]
            n107 = Replace Array Subset(array=string[][] [["R charge (mhom)\t", "-", "NA", "-", "FAIL", "Résistance à une charge de -260.000000 A"]] ("Tableau"), new element #1=w331, index (row) #1=w319, index (col) #1=1 ("indice désactivé (col)"), new element #2=w324, index (row) #2=w319, index (col) #2=3 ("indice désactivé (col)"), new element #3=w320, index (row) #3=w319, index (col) #3=5 ("indice désactivé (col)")) -> (w353:string[][])
            n108 = Number To Decimal String(number=w342) -> (decimal integer string=w352:string)  [unwired: 1 in]
            n109 = Build Array(w352, "DCIR -" ("élément"), w339, w338, "NA" ("élément")) -> (w349:string[])
            n110 = Replace Array Subset(array=w353, new element=w336, index (col)=4 ("indice désactivé (col)")) -> (w354:string[][])  [unwired: 1 in]
            n111 = call "HTML_Table_Head.vi"("entrée d'erreur (pas d'erreur)"=w332, "Tableau"=w349, "chaîne en entrée"=w345) -> ("sortie d'erreur"=w350:errorcluster, "result string"=w351:string)  [unwired: 7 in]
            n112 = call "HTML_Table_Data.vi"("entrée d'erreur (pas d'erreur)"=w350, "Tableau"=w354, "chaîne en entrée"=w351) -> ("sortie d'erreur"=w344:errorcluster, "result string"=w335:string)  [unwired: 7 in]
          }
          frame "DCIR+" {
            w474 = 0 ("indice désactivé (col)")
            # "29/08/2022_09:33:29;DCIR-;DCIR avec une charge à -260.0000 A donne ; 1.8140 mhom ;"
            n113 = Index Array(array=w492) -> (element #4=w485:string)  [unwired: 4 in, 3 out]
            n114 = Select(t="Résistance à une charge de +260.000000 A", s=w470, f="Résistance à une charge de +174.000000 A") -> (s? t:f=w471:string)
            n115 = xnode "Rechercher une expression régulière"("chaîne en entrée"=w485, "expression régulière"="[0-9|.]+") -> ("toute l'expression"=w482:string)  [unwired: 4 in, 4 out]
            n116 = Fract/Exp String To Number(string=w482) -> (number=w480:dbl)  [unwired: 3 in, 1 out]
            n117 = Increment(x=w494) -> (x+1=w493:i32)
            n118 = Less Or Equal?(x=w480, y=w477) -> (x <= y?=w479:bool)
            n119 = Number To Fractional String(number=w477, precision (6)=i16 3 ("précision (6)")) -> (F-format string=w475:string)  [unwired: 2 in]
            n120 = Build Array(w479) -> (w491:bool[])
            n121 = call <userlib>:"DataCell_NbPASSFAIL_Bool.vi"("Tableau en entrée"=w491) -> ("Chaîne"=w489:string, "Chaîne 2"=w490:string, "Tableau en sortie"=w487:string[])  [unwired: 8 in]
            n122 = Number To Decimal String(number=w493) -> (decimal integer string=w503:string)  [unwired: 1 in]
            n123 = Replace Array Subset(array=string[][] [["R charge (mhom)\t", "-", "NA", "-", "FAIL", "Résistance à une charge de +260.000000 A"]] ("Tableau"), new element #1=w482, index (row) #1=w474, index (col) #1=1 ("indice désactivé (col)"), new element #2=w475, index (row) #2=w474, index (col) #2=3 ("indice désactivé (col)"), new element #3=w471, index (row) #3=w474, index (col) #3=5 ("indice désactivé (col)")) -> (w504:string[][])
            n124 = Build Array(w503, "DCIR +" ("élément"), w490, w489, "NA" ("élément")) -> (w500:string[])
            n125 = Replace Array Subset(array=w504, new element=w487, index (col)=4 ("indice désactivé (col)")) -> (w505:string[][])  [unwired: 1 in]
            n126 = call "HTML_Table_Head.vi"("entrée d'erreur (pas d'erreur)"=w483, "Tableau"=w500, "chaîne en entrée"=w496) -> ("sortie d'erreur"=w501:errorcluster, "result string"=w502:string)  [unwired: 7 in]
            n127 = call "HTML_Table_Data.vi"("entrée d'erreur (pas d'erreur)"=w501, "Tableau"=w505, "chaîne en entrée"=w502) -> ("sortie d'erreur"=w495:errorcluster, "result string"=w486:string)  [unwired: 7 in]
          }
          frame "Test# 5 - predcir" {
            # "29/08/2022_09:32;Test# 5 - predcir;23.5000;23.5000;23.6000;23.6000;3.6304;3.6291;3.6291;3.6291;"
            n128 = call "Pv gen100 micro1.vi"("FluxStrIn"=w621, "Numin"=w622, "DeltaCell"=w630, "TempMin"=w635, "DeltaMv"=w631, "errin"=w629, "testlabel"="pré-DCIR" ("élément"), "Vmax"=w632, "tab ref"=string[][] [["t0 Cell1 Voltage(V)\t", "-", "NA", "NA", "FAIL", "Voltage cellule #1"], ["t0 Cell2 Voltage(V)\t", "", "NA", "NA", "FAIL", "Voltage cellule #2"], ["t0 Cell3 Voltage(V)\t", "", "NA", "NA", "FAIL", "Voltage cellule #3"], ["t0 Cell4 Voltage(V)\t", "", "NA", "NA", "FAIL", "Voltage cellule #4"], ["t0 Cell5 Voltage(V)\t", "", "NA", "NA", "FAIL", "Voltage cellule #5"], ["t0 Cell6 Voltage(V)\t", "", "NA", "NA", "FAIL", "Voltage cellule #6"], ["t0 Temp 1(C°)\t", "", "NA", "NA", "FAIL", "Température CTN #1"], ["t0 Temp 2(C°)\t", "", "NA", "NA", "FAIL", "Température CTN #2"], ["Delta Cell (mV)\t", "", "NA", "NA", "FAIL", "Ecart de tension cell (max-min)"], ["Delta temp (°C)\t", "", "NA", "NA", "FAIL", "Ecart de température cell (max-min)"]] ("Tableau"), "Vmin"=w633, "ligne à traiter"=w623, "TempMax"=w634, "3P4S?"=w620) -> ("result string"=w626:string, "Numout"=w627:i32, "errout"=w628:errorcluster)  [unwired: 4 in]
          }
          frame "Test# 6 - postdcir" {
            # "29/08/2022_09:32;Test# 5 - predcir;23.5000;23.5000;23.6000;23.6000;3.6304;3.6291;3.6291;3.6291;"
            n129 = call "Pv gen100 micro1.vi"("FluxStrIn"=w650, "Numin"=w647, "DeltaCell"=w639, "TempMin"=w643, "DeltaMv"=w638, "errin"=w649, "testlabel"="post-DCIR" ("élément"), "Vmax"=w640, "tab ref"=string[][] [["t2 Cell1 Voltage(V)\t", "-", "NA", "NA", "FAIL", "Voltage cellule #1"], ["t2 Cell2 Voltage(V)\t", "", "NA", "NA", "FAIL", "Voltage cellule #2"], ["t2 Cell3 Voltage(V)\t", "", "NA", "NA", "FAIL", "Voltage cellule #3"], ["t2 Cell4 Voltage(V)\t", "", "NA", "NA", "FAIL", "Voltage cellule #4"], ["t2 Cell5 Voltage(V)\t", "", "NA", "NA", "FAIL", "Voltage cellule #5"], ["t2 Cell6 Voltage(V)\t", "", "NA", "NA", "FAIL", "Voltage cellule #6"], ["t2 Temp 1(C°)\t", "", "NA", "NA", "FAIL", "Température CTN #1"], ["t2 Temp 2(C°)\t", "", "NA", "NA", "FAIL", "Température CTN #2"], ["Delta Cell (mV)\t", "", "NA", "NA", "FAIL", "Ecart de tension cell (max-min)"], ["Delta temp (°C)\t", "", "NA", "NA", "FAIL", "Ecart de température cell (max-min)"]] ("Tableau"), "Vmin"=w641, "ligne à traiter"=w645, "TempMax"=w642, "3P4S?"=w636) -> ("result string"=w644:string, "Numout"=w646:i32, "errout"=w648:errorcluster)  [unwired: 4 in]
          }
          frame "Test# 5.5 - intradcir" {
            # "29/08/2022_09:32;Test# 5 - predcir;23.5000;23.5000;23.6000;23.6000;3.6304;3.6291;3.6291;3.6291;"
            n130 = expression code="x+0.3"(w655) -> (w654:dbl)
            n131 = expression code="x-0.3"(w656) -> (w657:dbl)
            n132 = call "Pv gen100 micro1.vi"("FluxStrIn"=w664, "Numin"=w665, "DeltaCell"=w667, "TempMin"=w669, "DeltaMv"=w652, "errin"=w666, "testlabel"="intra-DCiR" ("élément"), "Vmax"=w654, "tab ref"=string[][] [["t1 Cell1 Voltage(V)\t", "-", "NA", "NA", "FAIL", "Voltage cellule #1"], ["t1 Cell2 Voltage(V)\t", "", "NA", "NA", "FAIL", "Voltage cellule #2"], ["t1 Cell3 Voltage(V)\t", "", "NA", "NA", "FAIL", "Voltage cellule #3"], ["t1 Cell4 Voltage(V)\t", "", "NA", "NA", "FAIL", "Voltage cellule #4"], ["t1 Cell5 Voltage(V)\t", "", "NA", "NA", "FAIL", "Voltage cellule #5"], ["t1 Cell6 Voltage(V)\t", "", "NA", "NA", "FAIL", "Voltage cellule #6"], ["t1 Temp 1(C°)\t", "", "NA", "NA", "FAIL", "Température CTN #1"], ["t1 Temp 2(C°)\t", "", "NA", "NA", "FAIL", "Température CTN #2"], ["Delta Cell (mV)\t", "", "NA", "NA", "FAIL", "Ecart de tension cell (max-min)"], ["Delta temp (°C)\t", "", "NA", "NA", "FAIL", "Ecart de température cell (max-min)"]] ("Tableau"), "Vmin"=w657, "ligne à traiter"=w662, "TempMax"=w668, "3P4S?"=w653) -> ("result string"=w661:string, "Numout"=w660:i32, "errout"=w659:errorcluster)  [unwired: 4 in]
          }
          frame "NULL", Default {
            # "NULL"
          }
        }
      }
    }
    frame Error {
    }
  }
  n133 = Search and Replace String(replace all?=TRUE ("tout remplacer ? (F)"), input string=w75, search string="<td class=\"core1 testpass\">FAIL</td>" ("chaîne recherchée"), replace string="<td class=\"core1 testfail\">FAIL</td>" ("chaîne de remplacement (\"\")"), error in=w73) -> (result string=w59:string, number of replacements=w54:i32, error out=w70:errorcluster)  [unwired: 3 in, 1 out]
  n134 = Search and Replace String(replace all?=TRUE ("tout remplacer ? (F)"), input string=w59, search string="<td class=\"core1 testpass\">PASS</td>" ("chaîne recherchée"), error in=w70) -> (number of replacements=w62:i32, error out=w66:errorcluster)  [unwired: 4 in, 2 out]
  "nombre de remplacements" <- w62
  n135 = Number To Decimal String(number=w62) -> (decimal integer string=w61:string)  [unwired: 1 in]
  n136 = Number To Decimal String(number=w54) -> (decimal integer string=w60:string)  [unwired: 1 in]
  n137 = Search and Replace String(input string=w59, search string="<!--NBTESTOK-->" ("chaîne recherchée"), replace string=w61, error in=w66) -> (result string=w67:string, error out=w65:errorcluster)  [unwired: 4 in, 2 out]
  n138 = Equal To 0?(x=w54) -> (x = 0?=w15:bool)
  n139 = Search and Replace String(input string=w67, search string="<!--NBTESTKO-->" ("chaîne recherchée"), replace string=w60, error in=w65) -> (result string=w47:string, error out=w53:errorcluster)  [unwired: 4 in, 2 out]
  n140 = Search and Replace String(input string=w47, search string="Résultat du test :\t</td><td class=\"resume5\" colspan=\"3\"><div><span style=\"float:left\" id=\"result\"><font color=\"green\"><b>PASS</b>", replace string="Résultat du test :\t</td><td class=\"resume5\" colspan=\"3\"><div><span style=\"float:left\" id=\"result\"><font color=\"red\"><b>FAIL</b>", error in=w53) -> (result string=w48:string, error out=w52:errorcluster)  [unwired: 4 in, 2 out]
  n141 = Select(t=w47, s=w15, f=w48) -> (s? t:f=w49:string)
  "Chaîne" <- w49
  n142 = Not Equal?(x=w10, y=path "") -> (x != y?=w12:bool)
  n143 = Open/Create/Replace File(file path (use dialog)=w76, error in=w52, operation (0:open)=w58) -> (refnum out=w82:refnum<file>, error out=w84:errorcluster)  [unwired: 3 in, 1 out]
  n144 = case shown="Vrai" w12 {
    tunnel: w58 -> [_ w680]
    tunnel: w10 -> [_ w679]
    tunnel: w52 -> [_ w678]
    tunnel: w49 -> [_ w677]
    tunnel: [errorcluster {"status"=FALSE, "code"=0, "source"=""} ("error out") w676] -> w17
    frame False {
    }
    frame True {
      n145 = Open/Create/Replace File(file path (use dialog)=w679, error in=w678, operation (0:open)=w680) -> (refnum out=w681:refnum<file>, error out=w683:errorcluster)  [unwired: 3 in, 1 out]
      n146 = Write to Text File(file (use dialog)=w681, text=w677, error in=w683) -> (refnum out=w682:refnum<file>, error out=w684:errorcluster)  [unwired: 1 in, 1 out]
      n147 = Close File(refnum=w682, error in=w684) -> (error out=w676:errorcluster)  [unwired: 1 out]
    }
  }
  n148 = Write to Text File(file (use dialog)=w82, text=w49, error in=w84) -> (refnum out=w83:refnum<file>, error out=w85:errorcluster)  [unwired: 1 in, 1 out]
  n149 = Close File(refnum=w83, error in=w85) -> (error out=w16:errorcluster)  [unwired: 1 out]
  n150 = Merge Errors(w16, w17) -> (w14:errorcluster)
  "sortie d'erreur" <- w14
  n151 = Compound Arithmetic op=AND ("Opérateur arithmétique")(w15, invert w14) -> (→"tout bon":bool)
